vi "Create Outline.vi"(7 "3D Ribbon Property":T4={"General Property"={"Plot Name"="", "Coordinate System"=enum."Cartesian", "Opacity"=0.0}, "Projection Property"={"Draw XY"=FALSE, "Draw YZ"=FALSE, "Draw XZ"=FALSE}, "Plot Property"={"Draw Surface"=FALSE, "Color Ramp Cluster"={"Color Ramp Style"=enum."None", "Color Ramp Array"=[16711934, 393471, 57855, 4390754, 16449346, 16744722, 16711680], "Color Ramp Index"=[45, 91, 133, 175, 219, 255], "Interpolate?"=FALSE, "Logarithm?"=FALSE}, "Line Style"=enum."None", "Line Width"=0.0, "Line Color"=0, "Antialiasing"=FALSE}, "Ribbon Property"={"Ribbon Mode"=enum."Row", "Ribbon Width"=0.0}}, 8 "error in (no error)":errorcluster, 10 "Plot Representation In":T1, 11 "Plot Object In":refnum<vi>) -> (0 "error out":errorcluster, 2 "Plot Representation Out":T1, 3 "Plot Object Out":refnum<vi>, 4 "Outline Object Out":refnum<vi>)   [LabVIEW 2017, in "3D Ribbon.lvclass"]
uses:
  <vilib>/Math Plots/3D Math Plots/3D Ribbon/3D Ribbon/3D Ribbon.lvclass
  <vilib>/Math Plots/3D Math Plots/3D Ribbon/3D Ribbon/Typedef/3D Ribbon Property.ctl
  <vilib>/Math Plots/3D Math Plots/3D Plot/3D Plot/Typedef/Color Ramp Cluster.ctl
  <vilib>/Math Plots/3D Math Plots/3D Plot/3D Plot/Typedef/Line Type.ctl
  <vilib>/Math Plots/3D Math Plots/3D Plot/3D Plot/Typedef/Plot Representation.ctl
  <vilib>/Math Plots/3D Math Plots/3D Plot/3D Plot/Typedef/Range Clusters.ctl
  <vilib>/Math Plots/3D Math Plots/3D Plot/3D Plot/Typedef/Mesh Data.ctl
  <vilib>/picture/3D Picture Control/NI_3D Picture Control.lvlib
  <vilib>/Math Plots/3D Math Plots/3D Plot/3D Plot/3D Plot.lvclass
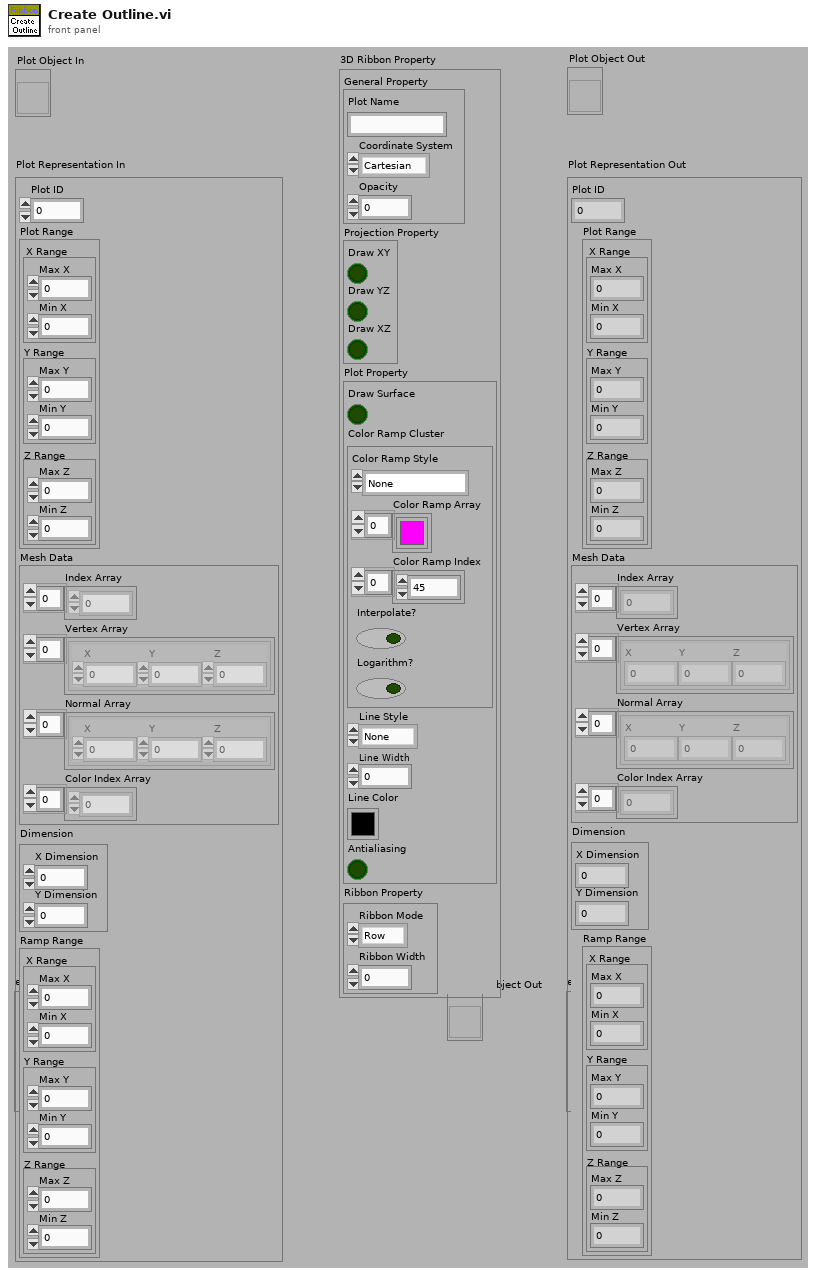
[diagram p1: front panel]
types:
  T1 = typedef "3D Plot.lvclass/Plot Representation.ctl" = cluster{"Plot ID":i32, "Plot Range":T2, "Mesh Data":T3, "Dimension":cluster{"X Dimension":i32, "Y Dimension":i32}, "Ramp Range":T2}
  T2 = typedef "3D Plot.lvclass/Range Clusters.ctl" = cluster{"X Range":cluster{"Max X":sgl, "Min X":sgl}, "Y Range":cluster{"Max Y":sgl, "Min Y":sgl}, "Z Range":cluster{"Max Z":sgl, "Min Z":sgl}}
  T3 = typedef "3D Plot.lvclass/Mesh Data.ctl" = cluster{"Index Array":u32[], "Vertex Array":cluster{"X":sgl, "Y":sgl, "Z":sgl}[], "Normal Array":cluster{"X":sgl, "Y":sgl, "Z":sgl}[], "Color Index Array":i32[]}
  T4 = typedef "3D Ribbon.lvclass/3D Ribbon Property.ctl" = cluster{"General Property":cluster{"Plot Name":string, "Coordinate System":enum16{"Cartesian", "Cylindrical", "Spherical"}, "Opacity":sgl}, "Projection Property":cluster{"Draw XY":bool, "Draw YZ":bool, "Draw XZ":bool}, "Plot Property":cluster{"Draw Surface":bool, "Color Ramp Cluster":T5, "Line Style":T6, "Line Width":sgl, "Line Color":u32, "Antialiasing":bool}, "Ribbon Property":cluster{"Ribbon Mode":enum16{"Row", "Column"}, "Ribbon Width":sgl}}
  T5 = typedef "3D Plot.lvclass/Color Ramp Cluster.ctl" = cluster{"Color Ramp Style":enum16{"None", "Shaded", "Color spectrum", "Grey scale", "Custom"}, "Color Ramp Array":u32[], "Color Ramp Index":i32[], "Interpolate?":bool, "Logarithm?":bool}
  T6 = typedef "3D Plot.lvclass/Line Type.ctl" = enum16{"None", "Solid", "Dash", "Dot", "Dash Dot"}
  T7 = enum16{"Points", "Lines", "Line Strip", "Line Loop", "Triangles", "Triangle Strip", "Triangle Fan", "Quads", "Quad Strip", "Polygon"}
  T8 = enum16{"Overall", "Per Primitive", "Per Vertex", "Binding Off"}
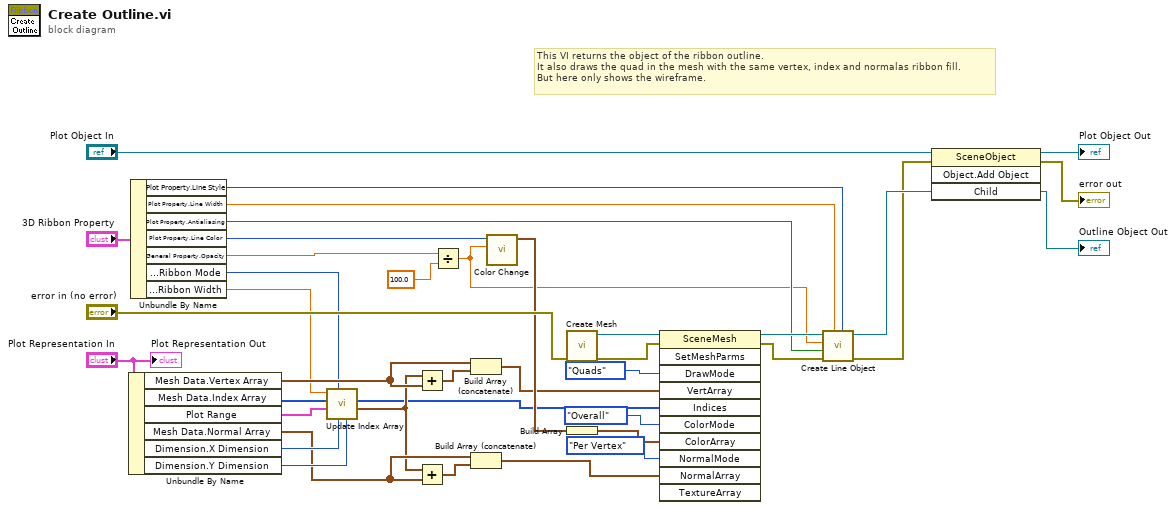
[diagram p0: block diagram]
diagram:
  # "This VI returns the object of the ribbon outline.\nIt also draws the quad in the mesh with the same vertex, index and normalas ribbon fill.\nBut here only shows the wireframe."
  n1 = Unbundle By Name("Plot Representation In") -> ("Mesh Data.Vertex Array"=w9:cluster{"X":sgl, "Y":sgl, "Z":sgl}[], "Mesh Data.Index Array"=w14:u32[], "Plot Range"=w8:T2, "Mesh Data.Normal Array"=w7:cluster{"X":sgl, "Y":sgl, "Z":sgl}[], "Dimension.X Dimension"=w13:i32, "Dimension.Y Dimension"=w12:i32)
  n2 = Unbundle By Name("3D Ribbon Property") -> ("Plot Property.Line Style"=w21:T6, "Plot Property.Line Width"=w22:sgl, "Plot Property.Antialiasing"=w19:bool, "Plot Property.Line Color"=w27:u32, "General Property.Opacity"=w20:sgl, "Ribbon Property.Ribbon Mode"=w2:enum16{"Row", "Column"}, "Ribbon Property.Ribbon Width"=w3:sgl)
  n3 = call <vilib>:"Update Index Array.vi"("Y Dimension"=w12, "X Dimension"=w13, "Ribbon Mode"=w2, "Plot Range"=w8, "Index Array Input"=w14, "Ribbon Width"=w3) -> ("Point Offset"=w6:cluster{"X":sgl, "Y":sgl, "Z":sgl}, "Index Array Output"=w1:u32[])  [unwired: 2 in, 2 out]
  n4 = Add(x=w6, y=w9) -> (x+y=w10:cluster{"X":sgl, "Y":sgl, "Z":sgl}[])
  n5 = Add(x=w6, y=w7) -> (x+y=w11:cluster{"X":sgl, "Y":sgl, "Z":sgl}[])
  n6 = Divide(x=w20, y=sgl 100.0) -> (x/y=w18:sgl)
  n7 = Build Array (concatenate)(w9, w10) -> (w5:cluster{"X":sgl, "Y":sgl, "Z":sgl}[])
  n8 = Build Array (concatenate)(w7, w11) -> (w4:cluster{"X":sgl, "Y":sgl, "Z":sgl}[])
  n9 = call <vilib>:"Color Change.vi"("Alpha"=w18, "Color"=w27) -> ("RGBA"=w28:cluster{"R":sgl, "G":sgl, "B":sgl, "A":sgl})  [unwired: 9 out]
  n10 = call <vilib>:"Create Mesh.vi"("error in (no error)"="error in (no error)") -> ("error out"=w33:errorcluster, "New Mesh Refnum"=w34:refnum<vi>)  [unwired: 9 out]
  n11 = Build Array(w28) -> (w31:cluster{"R":sgl, "G":sgl, "B":sgl, "A":sgl}[])
  n12 = invoke class="SceneMesh" method="SetMeshParms"(reference=w34, error in=w33, "DrawMode"=T7."Quads" ("Draw Mode"), "VertArray"=w5, "Indices"=w1, "ColorMode"=T8."Overall" ("Color Binding Mode"), "ColorArray"=w31, "NormalMode"=T8."Per Vertex" ("Normal Binding Mode"), "NormalArray"=w4) -> (reference out=w24:refnum<vi>, error out=w23:errorcluster)  [unwired: 2 in, 9 out]
  n13 = call <vilib>:"Create Line Object.vi"("Line Style"=w21, "Line Width"=w22, "error in (no error)"=w23, "Antialiasing"=w19, "Alpha"=w18, "Mesh Ref In"=w24) -> ("error out"=w16:errorcluster, "Object Ref Out"=w17:refnum<vi>)  [unwired: 4 out]
  n14 = invoke class="SceneObject" method="Object.Add Object"(reference="Plot Object In", error in=w16, "Child"=w17) -> (reference out=→"Plot Object Out":refnum<vi>, error out=→"error out":errorcluster, "Child"=→"Outline Object Out":refnum<vi>)  [unwired: 1 in, 1 out]
  "Plot Representation Out" <- "Plot Representation In"
